vi "Stop Message.vi"(8 "error in (no error)":errorcluster, 11 "Pump Controller in":refnum<class "Pump Controller.lvclass">) -> (0 "error out":errorcluster, 2 "Stop Message":T1, 3 "Pump Controller out":refnum<class "Pump Controller.lvclass">)   [LabVIEW 2020, in "Pump Controller.lvclass"]
uses:
  Pump Controller.lvclass
  <userlib>/RxnRover/DynamicReentrant/src/Type Defs/Message.ctl
  <userlib>/RxnRover/DynamicReentrant/Dynamic Reentrant.lvlib
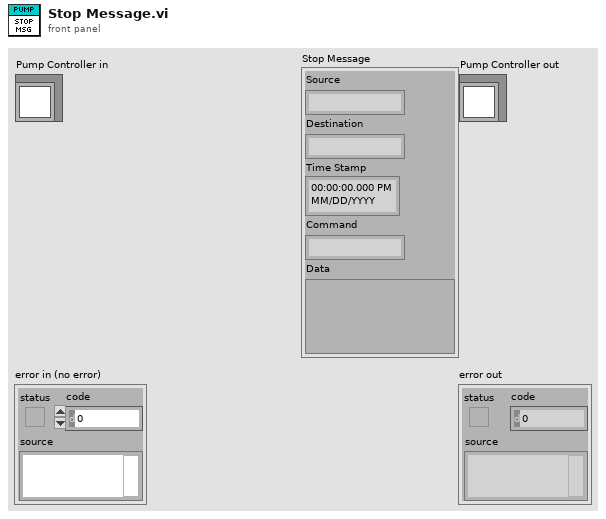
[diagram p1: front panel]
types:
  T1 = typedef "Dynamic Reentrant.lvlib/Message.ctl" = cluster{"Source":string, "Destination":string, "Time Stamp":timestamp, "Command":string, "Data":variant}
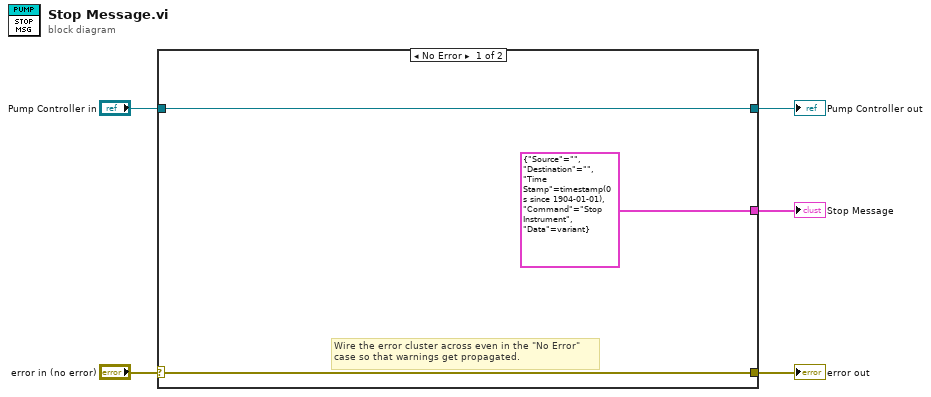
[diagram p0: block diagram]
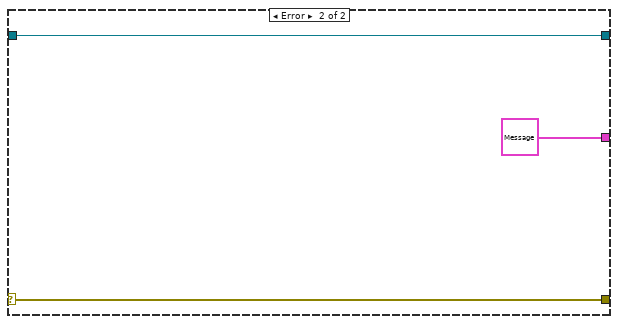
[diagram p2: hidden frame]
diagram:
  n1 = case shown="No Error" "error in (no error)" {
    selector: "error in (no error)" -> [w7 w11]
    tunnel: [w7 w11] -> w3
    tunnel: [w8 w10] -> w1
    tunnel: "Pump Controller in" -> [w8 w10]
    tunnel: [T1 {"Source"="", "Destination"="", "Time Stamp"=timestamp(0 s since 1904-01-01), "Command"="Stop Instrument", "Data"=variant} ("Message") T1 {"Source"="", "Destination"="", "Time Stamp"=timestamp(0 s since 1904-01-01), "Command"="", "Data"=variant} ("Message")] -> w2
    frame No Error {
      # "Wire the error cluster across even in the \"No Error\"\ncase so that warnings get propagated."
    }
    frame Error {
    }
  }
  "error out" <- w3
  "Pump Controller out" <- w1
  "Stop Message" <- w2
